vi "Run Function.vi"(0 "functionbase in":refnum<class "functionbase.lvclass">, 5 "Sub Functions":refnum<class "functionbase.lvclass">[](array[class]), 11 "error in (no error)":errorcluster) -> (4 "functionbase out":refnum<class "functionbase.lvclass">, 6 "Return":variant, 15 "error out":errorcluster)   [LabVIEW 2019, in "LSL.lvlib" / "functionbase.lvclass"]
uses:
  functionbase.lvclass
  functionbase.lvclass/functionbase.ctl
  properties/Read Indent#.vi
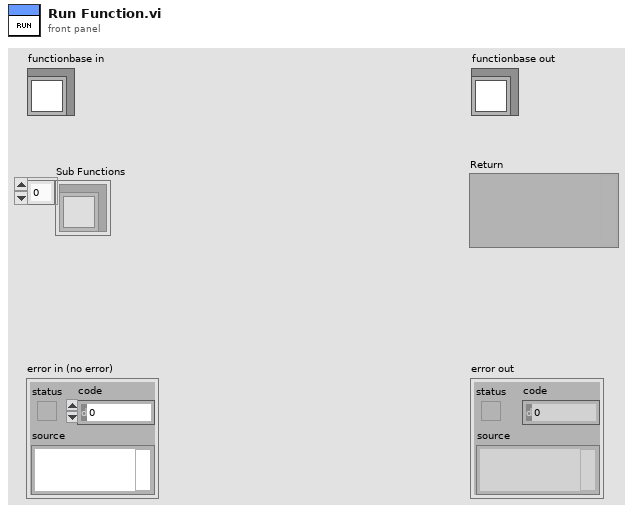
[diagram p1: front panel]
types:
  T1 = typedef "Function Indent Combo.ctl" = cluster{"Parent":refnum<class "functionbase.lvclass">, "Child":refnum<class "functionbase.lvclass">[]}
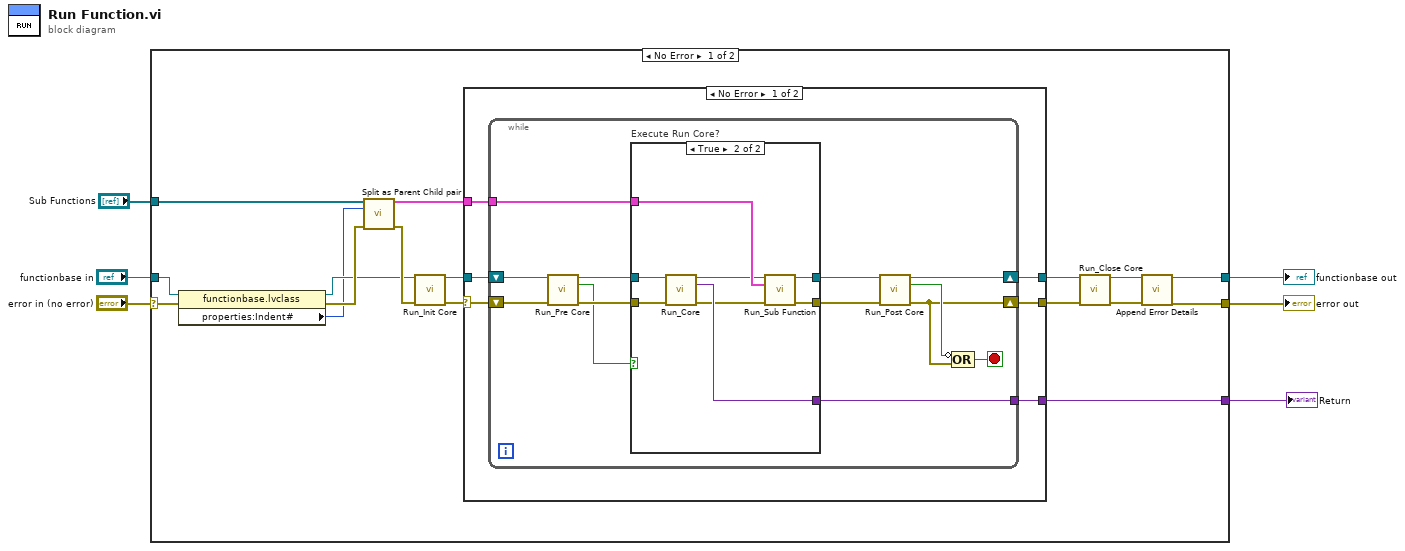
[diagram p0: block diagram]
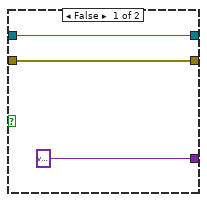
[diagram p2: hidden frame]
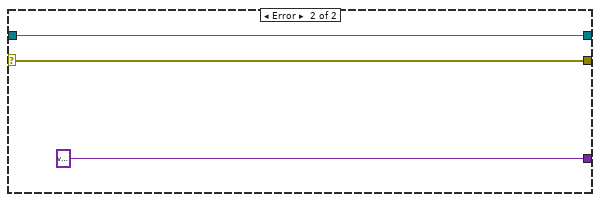
[diagram p3: hidden frame]
diagram:
  n1 = case shown="No Error" "error in (no error)" {
    selector: "error in (no error)" -> [w18 w58]
    tunnel: [w8 w58] -> w5
    tunnel: [w9 w57] -> w3
    tunnel: "functionbase in" -> [w19 w57]
    tunnel: "Sub Functions" -> [w21 _]
    tunnel: [w11 _] -> w1
    frame No Error {
      n2 = property class="functionbase.lvclass"(reference=w19, error in=w18) -> (reference out=w16:refnum<class "functionbase.lvclass">, error out=w17:errorcluster, "properties:Indent#"=w15:i64)
      n3 = call "Split as Parent Child pair.vi"("Functions"=w21, "Parent Indent"=w15, "error in (no error)"=w17) -> ("Parent Child Combo"=w14:T1[], "error out"=w20:errorcluster)  [unwired: 11 in]
      n4 = call-dynamic "Run_Init Core.vi"("functionbase in"=w16, "error in (no error)"=w20) -> ("functionbase out"=w22:refnum<class "functionbase.lvclass">, "error out"=w23:errorcluster)  [unwired: 12 in]
      n5 = case shown="No Error" w23 {
        selector: w23 -> [w29 w56]
        tunnel: w22 -> [w28 w55]
        tunnel: w14 -> [w27 _]
        tunnel: [w26 w55] -> w13
        tunnel: [w25 w56] -> w12
        tunnel: [w24 variant ("Return")] -> w11
        frame No Error {
          n6 = while {
            shift-right: [w35] -> w25
            shift-left: w29 -> [w42]
            shift-right: [w38] -> w26
            shift-left: w28 -> [w40]
            tunnel: w27 -> [w33]
            tunnel: [w34] -> w24
            stop <- w36 stop-if-true
            n7 = call-dynamic "Run_Pre Core.vi"("functionbase in"=w40, "error in (no error)"=w42) -> ("functionbase out"=w39:refnum<class "functionbase.lvclass">, "Execute Run Core?"=w30:bool, "error out"=w41:errorcluster)  [unwired: 11 in]
            n8 = case "Execute Run Core?" shown="True" w30 {
              tunnel: w41 -> [w44 w53]
              tunnel: w39 -> [w45 w52]
              tunnel: [variant ("Return") w51] -> w34
              tunnel: w33 -> [_ w50]
              tunnel: [w45 w48] -> w32
              tunnel: [w44 w47] -> w31
              frame False {
              }
              frame True {
                n9 = call-dynamic "Run_Core.vi"("functionbase in"=w52, "error in (no error)"=w53) -> ("functionbase out"=w49:refnum<class "functionbase.lvclass">, "Return"=w51:variant, "error out"=w46:errorcluster)  [unwired: 11 in]
                n10 = call-dynamic "Run_Sub Function.vi"("functionbase in"=w49, "Sub Function"=w50, "error in (no error)"=w46) -> ("functionbase out"=w48:refnum<class "functionbase.lvclass">, "error out"=w47:errorcluster)  [unwired: 11 in]
              }
            }
            n11 = call-dynamic "Run_Post Core.vi"("functionbase in"=w32, "error in (no error)"=w31) -> ("functionbase out"=w38:refnum<class "functionbase.lvclass">, "Go to Run Pre Core?"=w37:bool, "error out"=w35:errorcluster)  [unwired: 11 in]
            n12 = Compound Arithmetic op=OR(invert w37, w35) -> (w36:bool)
          }
        }
        frame Error {
        }
      }
      n13 = call-dynamic "Run_Close Core.vi"("functionbase in"=w13, "error in (no error)"=w12) -> ("functionbase out"=w10:refnum<class "functionbase.lvclass">, "error out"=w7:errorcluster)  [unwired: 12 in]
      n14 = call-dynamic "Append Error Details.vi"("functionbase in"=w10, "error in (no error)"=w7) -> ("functionbase out"=w9:refnum<class "functionbase.lvclass">, "error out"=w8:errorcluster)  [unwired: 12 in]
    }
    frame Error {
    }
  }
  "error out" <- w5
  "functionbase out" <- w3
  "Return" <- w1
